vi "LabVIEW to TOML.vi"(8 "error in (no error)":errorcluster, 11 "LV Value":variant) -> (0 "error out":errorcluster, 3 "TOML Value":T1)   [LabVIEW 2015, in "TOML.lvlib"]
uses:
  TOML.lvlib
  TOML Value.ctl
  Value.ctl
  Value Type.ctl
  Key-Value Pair.ctl
  <vilib>/Utility/Data Type/NI_Data Type.lvlib
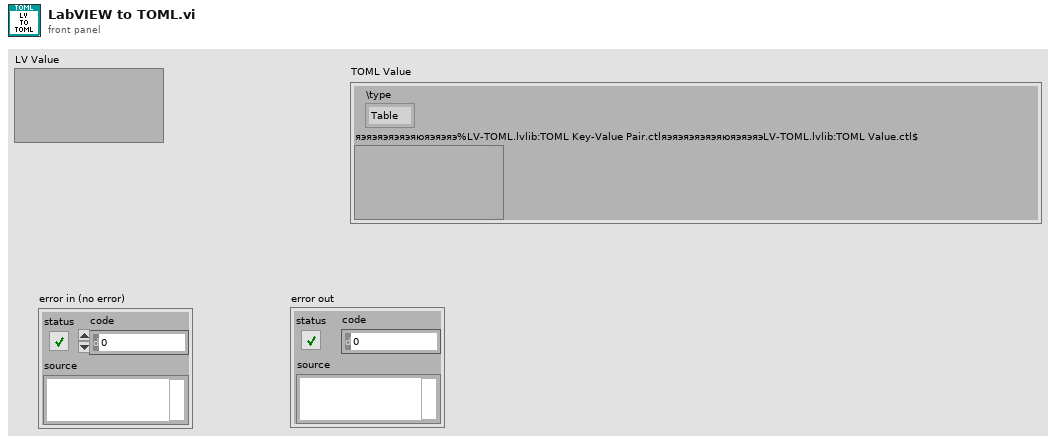
[diagram p1: front panel]
types:
  T1 = typedef "TOML.lvlib/TOML Value.ctl" = cluster{"\\type":enum16{"Table", "Array", "String", "Integer", "Float", "Boolean", "Offset Date-Time", "Local Date-Time", "Local Date", "Local Time"}, "яэяэяэяэяэяюяэяэяэ%LV-TOML.lvlib:TOML Key-Value Pair.ctlяэяэяэяэяэяюяэяэяэLV-TOML.lvlib:TOML Value.ctl$":variant}
  T2 = typedef "TOML.lvlib/Value.ctl" = cluster{"Type":T3, "Value":variant}
  T3 = typedef "TOML.lvlib/Value Type.ctl" = enum16{"Table", "Array", "String", "Integer", "Float", "Boolean", "Offset Date-Time", "Local Date-Time", "Local Date", "Local Time"}
  T4 = typedef "TOML.lvlib/Key-Value Pair.ctl" = cluster{"Key":string, "Value":T2}
  T5 = typedef "NI_Data Type.lvlib/Data Type.ctl" = enum8{"Invalid Type", "Void", "I8", "I16", "I32", "I64", "U8", "U16", "U32", "U64", "Single Float", "Double Float", "Extended Float", "Single Complex", "Double Complex", "Extended Complex", "Enum U8", "Enum U16", "Enum U32", "Enum U64", "Single Float With Unit", "Double Float With Unit", "Extended Float With Unit", "Single Complex with Unit", "Double Complex with Unit", "Extended Complex with Unit", "Boolean", "String", "Path", "Picture", "Tag", "Array", "Cluster", "Variant", "LV Variant", "Waveform", "Timestamp", "Digital Waveform", "Digital Data", "ExpressData", "Refnum", "External Data", "VI", "Poly VI", "LabVIEW Class Instance", "Fixed Point"}
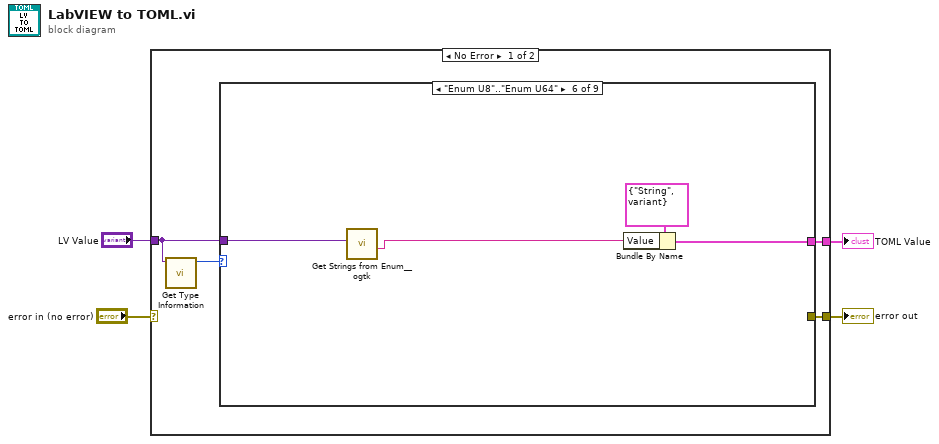
[diagram p0: block diagram]
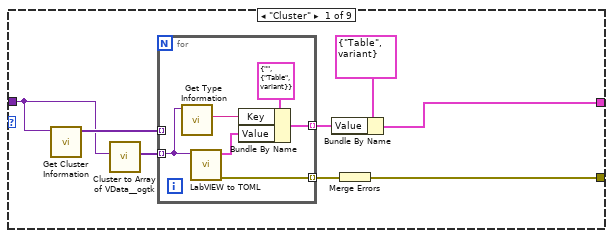
[diagram p2: hidden frame]
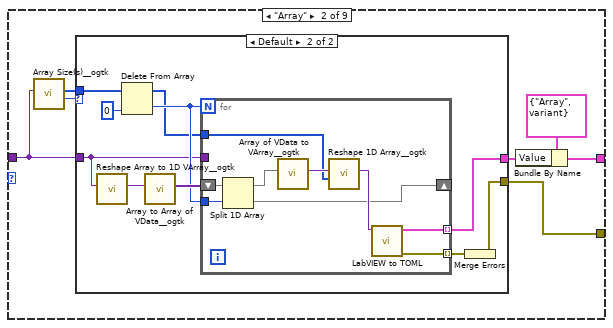
[diagram p3: hidden frame]
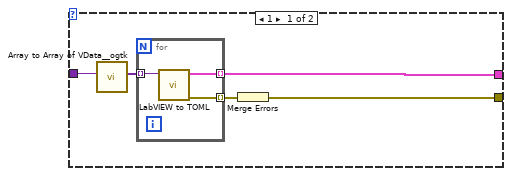
[diagram p4: hidden frame]
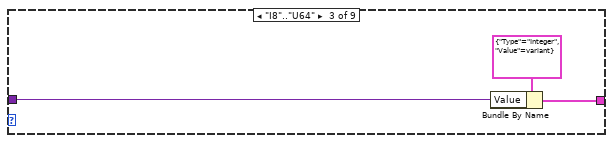
[diagram p5: hidden frame]
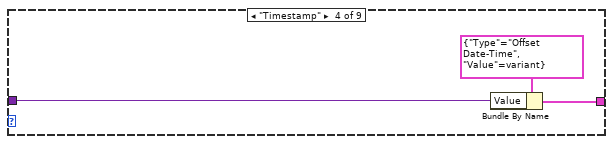
[diagram p6: hidden frame]
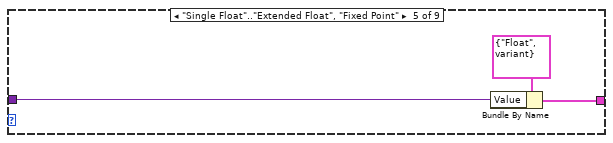
[diagram p7: hidden frame]
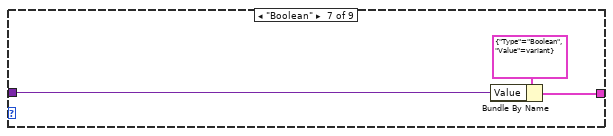
[diagram p8: hidden frame]
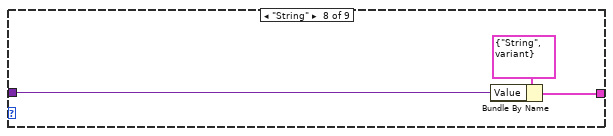
[diagram p9: hidden frame]
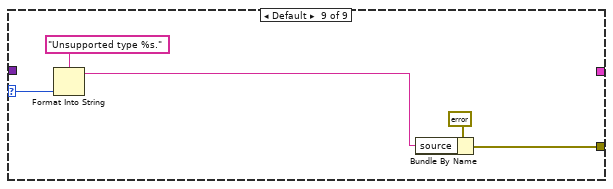
[diagram p10: hidden frame]
diagram:
  n1 = case shown="No Error" "error in (no error)" {
    selector: "error in (no error)" -> [_ w81]
    tunnel: "LV Value" -> [w6 _]
    tunnel: [w7 _] -> w3
    tunnel: [w5 w81] -> w1
    frame No Error {
      n2 = call <vilib>:"Get Type Information.vi"("Variant"=w6) -> ("Type"=w8:T5)  [unwired: 6 in, 4 out]
      n3 = case shown="\"Enum U8\"..\"Enum U64\"" w8 {
        selector: w8 -> [_ _ _ _ _ _ _ _ w80]
        tunnel: w6 -> [w15 w29 w57 w60 w63 w69 w70 w73 _]
        tunnel: [w11 w25 w59 w62 w65 w66 w72 w75 _] -> w7
        tunnel: [w9 w23 _ _ _ _ _ _ w77] -> w5
        frame "Cluster" {
          n4 = call <vilib>:"Get Cluster Information.vi"("Variant"=w15) -> ("Cluster Elements"=w16:variant[])  [unwired: 9 in, 1 out]
          n5 = call <userlib>:"Cluster to Array of VData__ogtk.vi"("Cluster"=w15) -> ("Array of VData"=w14:variant[])  [unwired: 9 in, 1 out]
          n6 = for {
            tunnel: w16 -> [_] mode=indexing
            tunnel: w14 -> [w22] mode=indexing
            tunnel: [w18] -> w13 mode=indexing
            tunnel: [w17] -> w10 mode=indexing
            n7 = call <vilib>:"Get Type Information.vi"("Variant"=w22) -> ("Name"=w20:string)  [unwired: 6 in, 4 out]
            n8 = call "LabVIEW to TOML.vi"("LV Value"=w22) -> ("error out"=w17:errorcluster, "TOML Value"=w19:T1)  [unwired: 9 in]
            n9 = Bundle By Name(cluster=T4 {"Key"="", "Value"={"Type"=enum."Table", "Value"=variant}} ("Key-Value Pair"), "Key"=w20, "Value"=w19) -> (w18:T4)
          }
          n10 = Bundle By Name(cluster=T2 {"Type"=enum."Table", "Value"=variant} ("Value"), "Value"=w13) -> (w11:T2)
          n11 = Merge Errors(w10) -> (w9:errorcluster)
        }
        frame "Array" {
          n12 = call <userlib>:"Array Size(s)__ogtk.vi"("Array"=w29) -> ("N dims"=w27:u32, "Size(s)"=w28:u32[])  [unwired: 8 in, 1 out]
          n13 = case shown="Default" w27 {
            tunnel: w29 -> [w34 w40]
            tunnel: w28 -> [_ w44]
            tunnel: [w32 w41] -> w26
            tunnel: [w30 w38] -> w23
            frame 1 {
              n14 = call <userlib>:"Array to Array of VData__ogtk.vi"("MultiD Array"=w34) -> ("1D Array of Variants"=w33:variant[])  [unwired: 9 in, 1 out]
              n15 = for {
                tunnel: w33 -> [w37] mode=indexing
                tunnel: [w36] -> w32 mode=indexing
                tunnel: [w35] -> w31 mode=indexing
                n16 = call "LabVIEW to TOML.vi"("LV Value"=w37) -> ("error out"=w35:errorcluster, "TOML Value"=w36:T1)  [unwired: 9 in]
              }
              n17 = Merge Errors(w31) -> (w30:errorcluster)
            }
            frame Default {
              n18 = call <userlib>:"Reshape Array to 1D VArray__ogtk.vi"("MultiD Array"=w40) -> ("1D VArray"=w47:variant)  [unwired: 8 in, 2 out]
              n19 = Delete From Array(array=w44, index=0) -> (deleted portion=w43:u32, array with subset deleted=w42:u32[])  [unwired: 1 in]
              n20 = call <userlib>:"Array to Array of VData__ogtk.vi"("MultiD Array"=w47) -> ("1D Array of Variants"=w46:variant[])  [unwired: 9 in, 1 out]
              n21 = for {
                N: w43 -> [_]
                tunnel: w40 -> [_]
                shift-right: [w49] -> _
                shift-left: w46 -> [w56]
                tunnel: w43 -> [w55]
                tunnel: w42 -> [w53]
                tunnel: [w51] -> w41 mode=indexing
                tunnel: [w48] -> w39 mode=indexing
                n22 = Split 1D Array(array=w56, index=w55) -> (first subarray=w50:variant[], second subarray=w49:variant[])
                n23 = call <userlib>:"Array of VData to VArray__ogtk.vi"("1D Array of VData"=w50) -> ("VArray"=w54:variant)  [unwired: 9 in, 1 out]
                n24 = call <userlib>:"Reshape 1D Array__ogtk.vi"("Size(s)"=w53, "1D Array"=w54) -> ("Reshaped VArray"=w52:variant)  [unwired: 8 in, 1 out]
                n25 = call "LabVIEW to TOML.vi"("LV Value"=w52) -> ("error out"=w48:errorcluster, "TOML Value"=w51:T1)  [unwired: 9 in]
              }
              n26 = Merge Errors(w39) -> (w38:errorcluster)
            }
          }
          n27 = Bundle By Name(cluster=T2 {"Type"=enum."Array", "Value"=variant} ("Value"), "Value"=w26) -> (w25:T2)
        }
        frame "I8".."U64" {
          n28 = Bundle By Name(cluster=T2 {"Type"=enum."Integer", "Value"=variant} ("Value"), "Value"=w57) -> (w59:T2)
        }
        frame "Timestamp" {
          n29 = Bundle By Name(cluster=T2 {"Type"=enum."Offset Date-Time", "Value"=variant} ("Value"), "Value"=w60) -> (w62:T2)
        }
        frame "Single Float".."Extended Float", "Fixed Point" {
          n30 = Bundle By Name(cluster=T2 {"Type"=enum."Float", "Value"=variant} ("Value"), "Value"=w63) -> (w65:T2)
        }
        frame "Enum U8".."Enum U64" {
          n31 = call <userlib>:"Get Strings from Enum__ogtk.vi"("Enum"=w69) -> ("String Value"=w67:string)  [unwired: 7 in, 3 out]
          n32 = Bundle By Name(cluster=T2 {"Type"=enum."String", "Value"=variant} ("Value"), "Value"=w67) -> (w66:T2)
        }
        frame "Boolean" {
          n33 = Bundle By Name(cluster=T2 {"Type"=enum."Boolean", "Value"=variant} ("Value"), "Value"=w70) -> (w72:T2)
        }
        frame "String" {
          n34 = Bundle By Name(cluster=T2 {"Type"=enum."String", "Value"=variant} ("Value"), "Value"=w73) -> (w75:T2)
        }
        frame Default {
          n35 = Format Into String(format string="Unsupported type %s.", w80) -> (resulting string=w76:string)  [unwired: 2 in, 1 out]
          n36 = Bundle By Name(cluster=errorcluster {"status"=TRUE, "code"=5001, "source"=""} ("error IO"), "source"=w76) -> (w77:errorcluster)
        }
      }
    }
    frame Error {
    }
  }
  "error out" <- w1
  "TOML Value" <- w3
